vi "Set Output State.vi"(8 "error in (no error)":errorcluster, 10 "Output State":bool, 11 "Simulated Water Level":refnum<class "Simulated Water Level.lvclass">) -> (0 "error out":errorcluster, 3 "Simulated Water Level":refnum<class "Simulated Water Level.lvclass">)   [LabVIEW 2018, in "Simulated Water Level.lvclass"]
doc: "This VI specifies the behavior of a level controller when the variable it is monitoring goes above the deadband or below the deadband. It is only invoked in the level controller class when the operation mode switches from one mode to another.\n\nIn this water level class, this VI specifies that when the water level falls below the deadband threshold, the valve opens. When the tank is refilled, the valve closes again."
uses:
  Simulated Water Level.lvclass
  Cooler Plug-Ins/Simulated Evaporative Cooler.lvclass/Simulation Data_Global.vi
  Cooler Plug-Ins/Simulated Evaporative Cooler.lvclass/Simulated Evaporative Cooler.lvclass
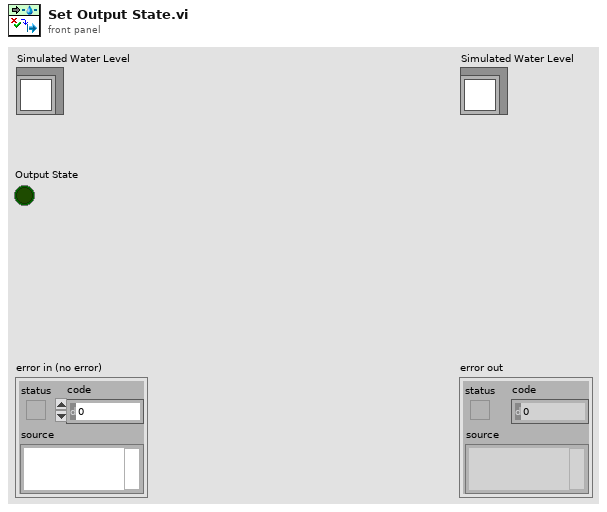
[diagram p1: front panel]
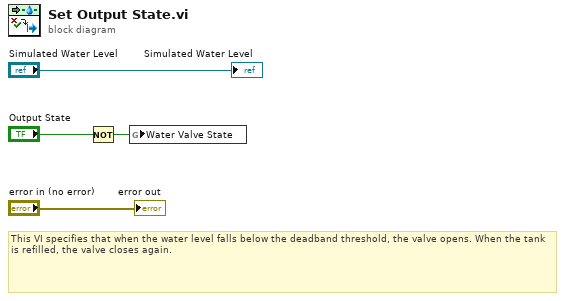
[diagram p0: block diagram]
diagram:
  # "This VI specifies that when the water level falls below the deadband threshold, the valve opens. When the tank is refilled, the valve closes again."
  n1 = Not(x="Output State") -> (.not. x?=w2:bool)
  n2 = global write "Simulation Data_Global.vi" "Water Valve State"(w2) -> ()
  "error out" <- "error in (no error)"
  "Simulated Water Level" <- "Simulated Water Level"
